vi "Deadzone 2 Sticks.vi"(0 "Input 1":dbl, 1 "Input 2":dbl, 2 "Input 3":dbl, 3 "Input 4":dbl, 4 "Input 5":dbl, 5 "Input 6":dbl, 6 "Input 7":dbl, 7 "Input 8":dbl, 13 "Deadzone":dbl) -> (20 "Output 1":dbl, 21 "Output 2":dbl, 22 "Output 3":dbl, 23 "Output 4":dbl, 24 "Output 5":dbl, 25 "Output 6":dbl, 26 "Output 7":dbl, 27 "Output 8":dbl)   [LabVIEW 2013]
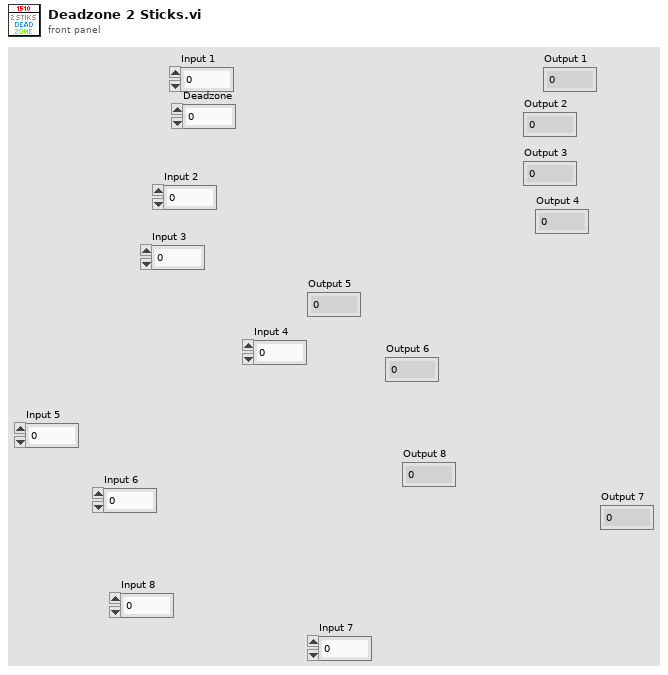
[diagram p1: front panel]
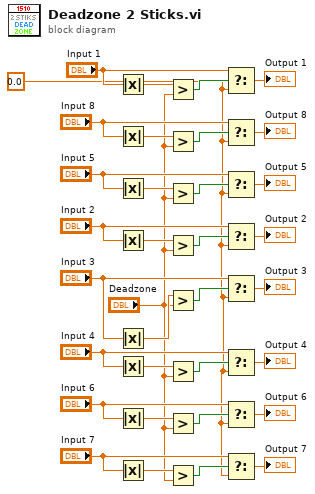
[diagram p0: block diagram]
diagram:
  w1 = 0.0 ("f")
  n1 = Absolute Value(x="Input 1") -> (abs(x)=w33:dbl)
  n2 = Absolute Value(x="Input 8") -> (abs(x)=w5:dbl)
  n3 = Absolute Value(x="Input 5") -> (abs(x)=w17:dbl)
  n4 = Absolute Value(x="Input 2") -> (abs(x)=w29:dbl)
  n5 = Absolute Value(x="Input 3") -> (abs(x)=w25:dbl)
  n6 = Absolute Value(x="Input 4") -> (abs(x)=w21:dbl)
  n7 = Absolute Value(x="Input 6") -> (abs(x)=w13:dbl)
  n8 = Absolute Value(x="Input 7") -> (abs(x)=w9:dbl)
  n9 = Greater?(x=w33, y="Deadzone") -> (0:w32:bool)
  n10 = Greater?(x=w5, y="Deadzone") -> (0:w4:bool)
  n11 = Greater?(x=w17, y="Deadzone") -> (0:w16:bool)
  n12 = Greater?(x=w29, y="Deadzone") -> (0:w28:bool)
  n13 = Greater?(x=w25, y="Deadzone") -> (0:w24:bool)
  n14 = Greater?(x=w21, y="Deadzone") -> (0:w20:bool)
  n15 = Greater?(x=w13, y="Deadzone") -> (0:w12:bool)
  n16 = Greater?(x=w9, y="Deadzone") -> (0:w8:bool)
  n17 = Select(t="Input 1", s=w32, f=w1) -> (s? t:f=→"Output 1":dbl)
  n18 = Select(t="Input 8", s=w4, f=w1) -> (s? t:f=→"Output 8":dbl)
  n19 = Select(t="Input 5", s=w16, f=w1) -> (s? t:f=→"Output 5":dbl)
  n20 = Select(t="Input 2", s=w28, f=w1) -> (s? t:f=→"Output 2":dbl)
  n21 = Select(t="Input 3", s=w24, f=w1) -> (s? t:f=→"Output 3":dbl)
  n22 = Select(t="Input 4", s=w20, f=w1) -> (s? t:f=→"Output 4":dbl)
  n23 = Select(t="Input 6", s=w12, f=w1) -> (s? t:f=→"Output 6":dbl)
  n24 = Select(t="Input 7", s=w8, f=w1) -> (s? t:f=→"Output 7":dbl)
